vi "Convert payload to float.vi"(0 "Byte1":u8=66 format="%.0x", 1 "Byte2":u8=51 format="%.0x", 2 "Byte3":u8=160 format="%.0x", 3 "Byte4":u8=18 format="%.0x", 4 "Invert":bool) -> (14 "FloatNumber":sgl)   [LabVIEW 2025]
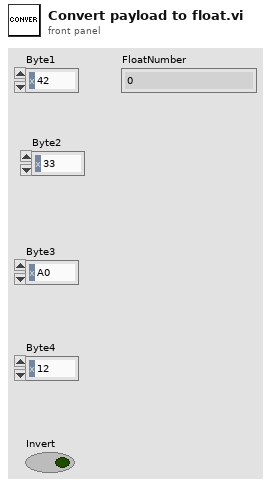
[diagram p1: front panel]
types:
  T1 = cluster{"ID":u32, "MSGTYPE":u8, "LEN":u8, "DATA[0]":u8, "DATA[1]":u8, "DATA[2]":u8, "DATA[3]":u8, "DATA[4]":u8, "DATA[5]":u8, "DATA[6]":u8, "DATA[7]":u8}
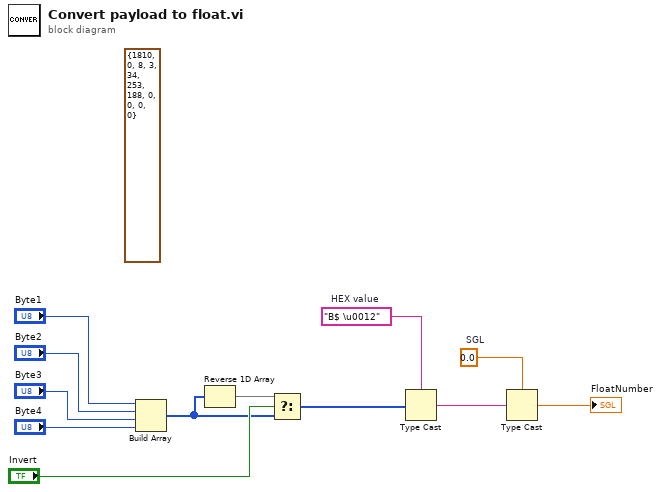
[diagram p0: block diagram]
diagram:
  (unwired) T1 {"ID"=1810, "MSGTYPE"=0, "LEN"=8, "DATA[0]"=3, "DATA[1]"=34, "DATA[2]"=253, "DATA[3]"=188, "DATA[4]"=0, "DATA[5]"=0, "DATA[6]"=0, "DATA[7]"=0} ("MessageBuffer")
  w12 = sgl 0.0  # SGL
  w10 = "B$ \u0012"  # HEX value
  n1 = Build Array("Byte1", "Byte2", "Byte3", "Byte4") -> (w2:u8[])
  n2 = Reverse 1D Array(array=w2) -> (reversed array=w1:u8[])
  n3 = Select(t=w1, s="Invert", f=w2) -> (s? t:f=w4:u8[])
  n4 = Type Cast(type=w10, x=w4) -> (*(type *) &x=w9:string)
  n5 = Type Cast(type=w12, x=w9) -> (*(type *) &x=→"FloatNumber":sgl)
